vi "AFT Estimate Maximum Step Size for FIR LMS.vi"(8 "error in (no error)":errorcluster, 10 "filter length":i32=128, 11 "x(n)":dbl[](array[numeric])) -> (0 "error out":errorcluster, 3 "maximum step size":dbl)   [LabVIEW 2017, in "NI_AdaptiveFilter.lvlib"]
doc: "Estimates the maximum step size for an adaptive filter that you create with the standard least mean squares (LMS) algorithm."
uses:
  <vilib>/addons/Adaptive Filters/NI_AdaptiveFilter.lvlib
  <vilib>/Analysis/baseanly.llb/Real Dot Product.vi
  <vilib>/Analysis/NI_AALBase.lvlib
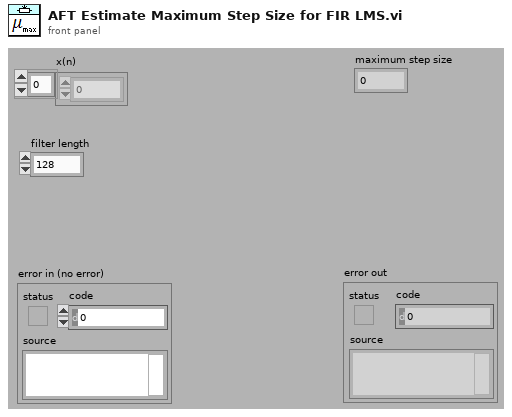
[diagram p1: front panel]
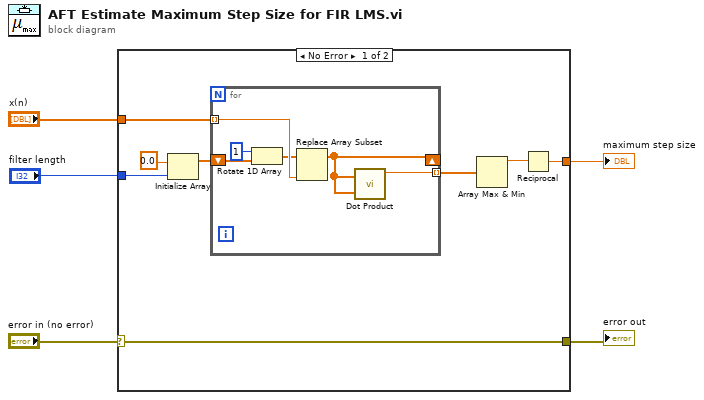
[diagram p0: block diagram]
diagram:
  n1 = case shown="No Error" "error in (no error)" {
    selector: "error in (no error)" -> [w13 w20]
    tunnel: "x(n)" -> [w9 _]
    tunnel: [w13 w20] -> w3
    tunnel: "filter length" -> [w8 _]
    tunnel: [w6 _] -> w1
    frame No Error {
      n2 = Initialize Array(0.0 ("element"), w8) -> (w11:dbl[])
      n3 = for {
        tunnel: w9 -> [w17] mode=indexing
        shift-right: [w15] -> _
        shift-left: w11 -> [w19]
        tunnel: [w14] -> w12 mode=indexing
        n4 = Rotate 1D Array(1:w19, 2:1 ("n")) -> (0:w16:dbl[])
        n5 = Replace Array Subset(array=w16, new element=w17) -> (w15:dbl[])  [unwired: 1 in]
        n6 = call-poly <vilib>:"Dot Product.vi"("Y Vector"=w15, "X Vector"=w15) -> ("X * Y"=w14:dbl)  [unwired: 1 out]
      }
      n7 = Array Max & Min(array=w12) -> (max value=w7:dbl)  [unwired: 3 out]
      n8 = Reciprocal(x=w7) -> (1/x=w6:dbl)
    }
    frame Error {
    }
  }
  "error out" <- w3
  "maximum step size" <- w1
